vi "Main.vi"() -> ()   [LabVIEW 2018]
uses:
  cluster_enum.ctl
  Notifier_control.ctl
  <vilib>/DAQmx/configure/timing.llb/DAQmx Timing (Sample Clock).vi
  <resource>/objmgr/daqmx.rc
panel:
  in  "C Module":T1=enum."Strain Card 1 Tared"
  in  "Stop 4":bool caption="Stop"
  in  "Card 2 Samples Per Loop":i32=100 caption="Numeric"
  in  "Tab Control":enum32{"Telemetry", "DAQ Settings"}(tab)
  in  "Save":bool
  in  "Test Name":string caption="String"
  out "Accel Card Rate":dbl caption="Numeric"
  in  "Card 2 Sample Rate Setpoint":dbl=100.0 caption="Numeric"
  in  "Card 1 Rate Setpoint":dbl=1000.0 caption="Numeric"
  out "Strain Card 1 Rate":dbl caption="Numeric"
  in  "Card 1 Samples Per Loop":i32=100 caption="Numeric"
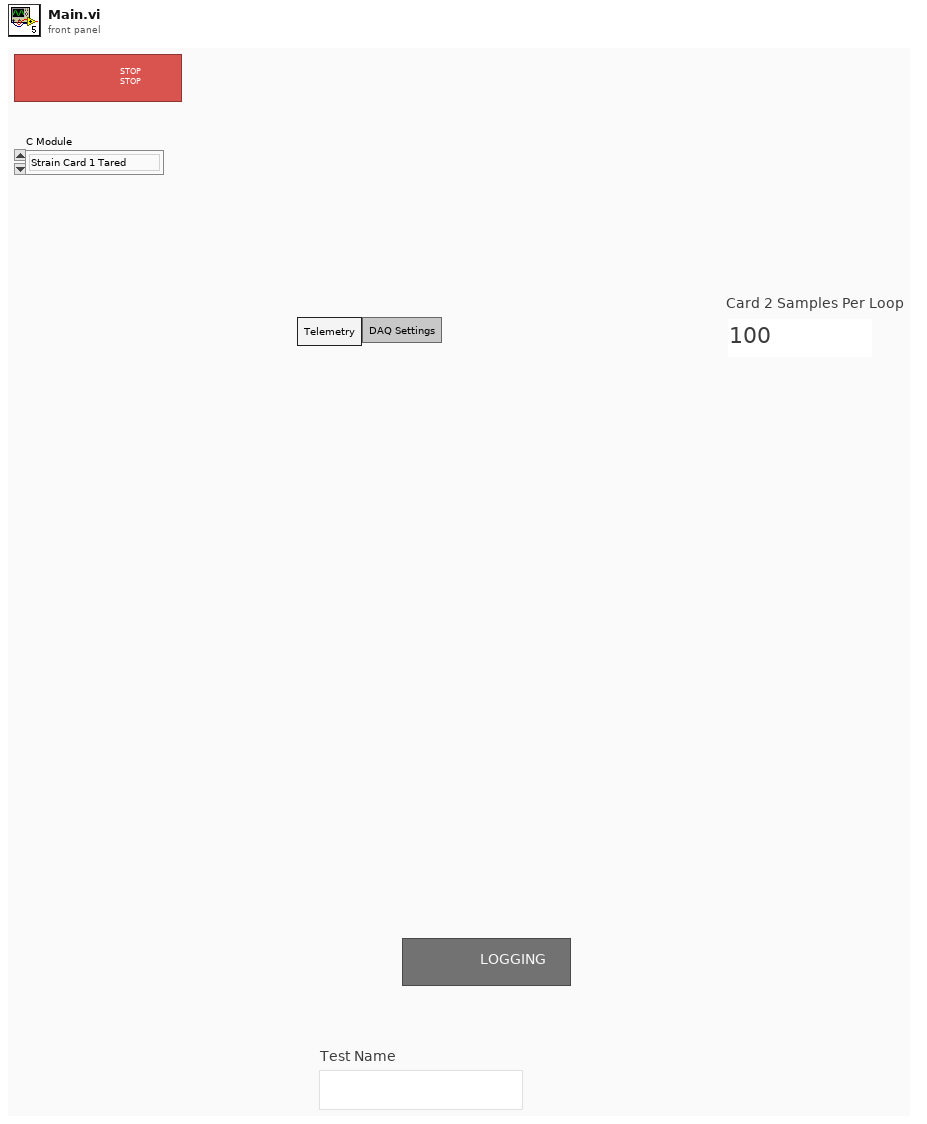
[diagram p1: front panel]
types:
  T1 = typedef "cluster_enum.ctl" = enum16{"Strain Card 2", "Strain Card 2 Tared", "Strain Card 1 Tared", "Strain Card 1", "Accel Card 1", "Accel Card 1 Tared", ""}
  T2 = typedef "Notifier_control.ctl" = enum16{"Quit", "Run", "Save"}
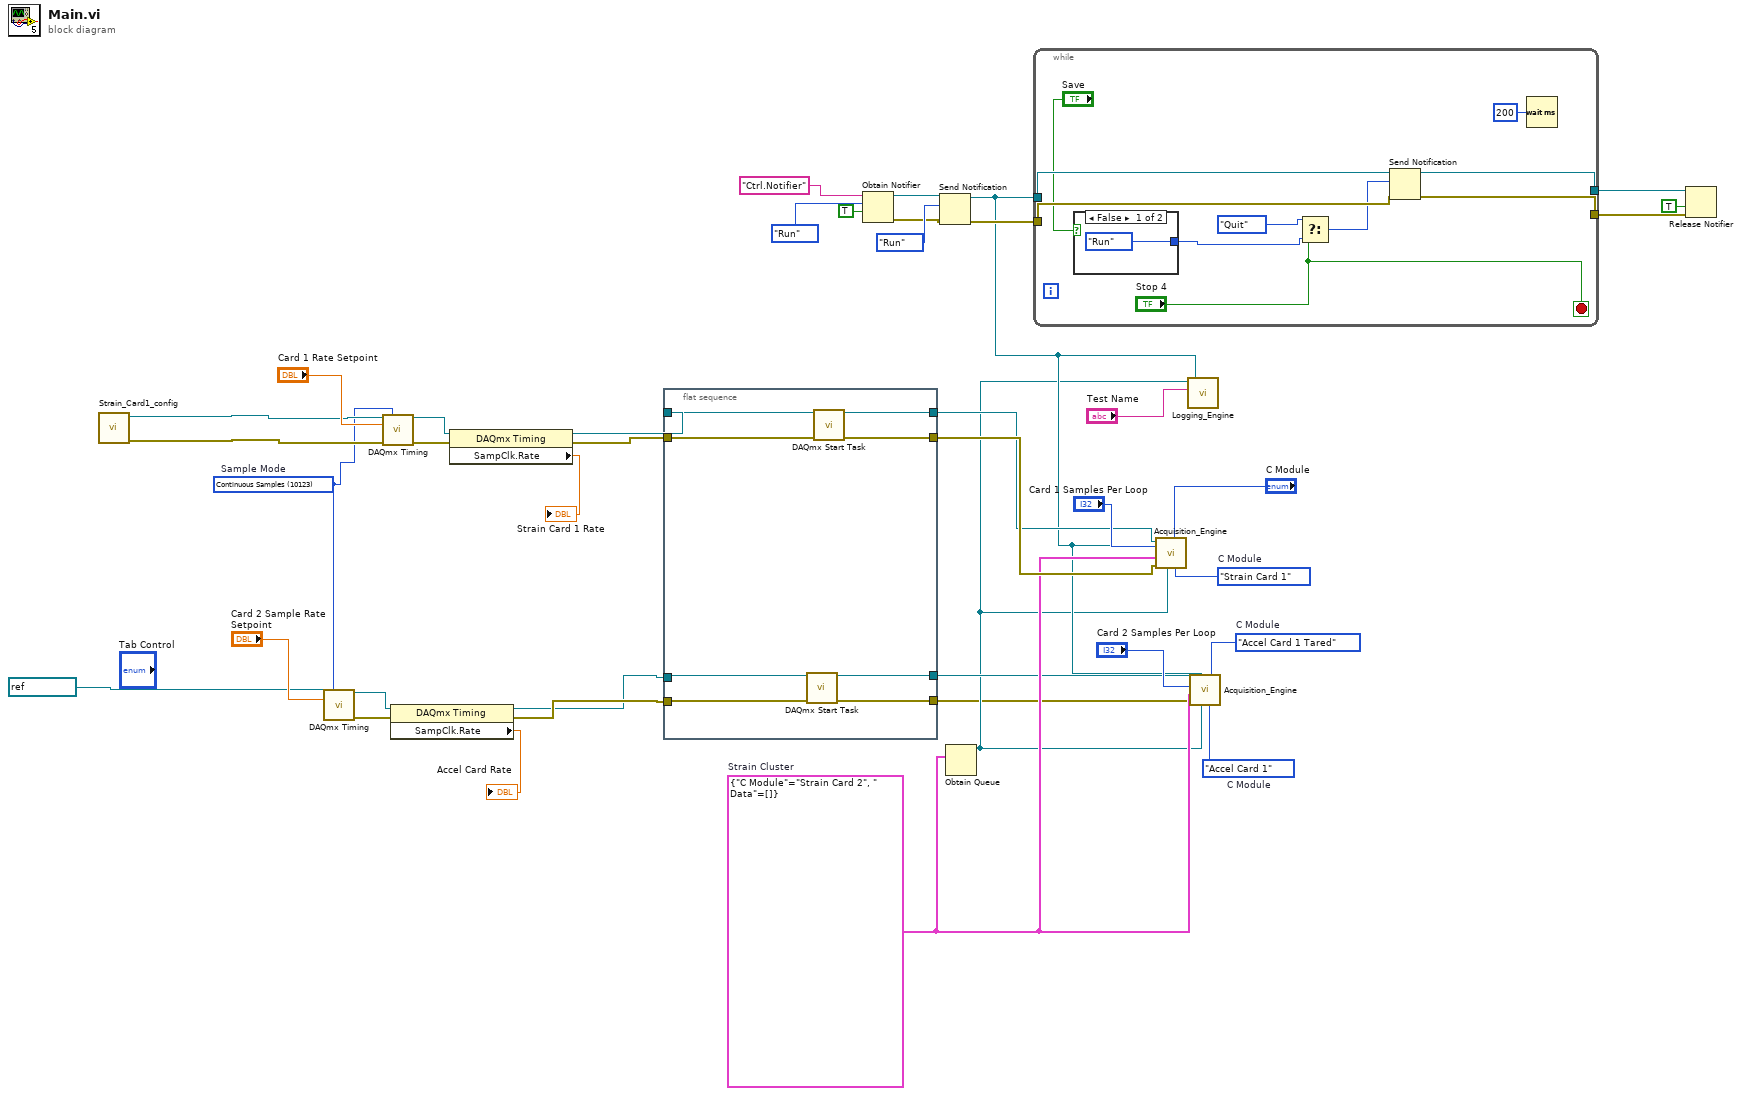
[diagram p0: block diagram]
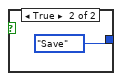
[diagram p2: hidden frame]
diagram:
  w2 = cluster_enum."Strain Card 1"  # C Module
  w3 = cluster_enum."Accel Card 1 Tared"  # C Module
  w4 = cluster_enum."Accel Card 1"  # C Module
  w10 = cluster{"C Module":T1, " Data":waveform(dbl)[]} {"C Module"=enum."Strain Card 2", " Data"=[]}  # Strain Cluster
  w26 = 10123 items=["Finite Samples"=10178, "Continuous Samples"=10123, "Hardware Timed Single Point"=12522]  # Sample Mode
  n1 = call "Strain_Card1_config.vi"() -> ("error out"=w33:errorcluster, "task out"=w34:refnum<k21>)  [unwired: 10 in]
  n2 = call-poly <vilib>:"DAQmx Timing.vi"("task/channels in"=refnum<k21> "Voltage", "sample mode"=w26, "rate"="Card 2 Sample Rate Setpoint") -> ("task out"=w32:refnum<k21>, "error out"=w31:errorcluster)  [unwired: 11 in]
  n3 = call-poly <vilib>:"DAQmx Timing.vi"("task/channels in"=w34, "sample mode"=w26, "rate"="Card 1 Rate Setpoint", "error in"=w33) -> ("task out"=w40:refnum<k21>, "error out"=w39:errorcluster)  [unwired: 10 in]
  n4 = property class="DAQmx Timing"(reference=w32, error in=w31) -> (reference out=w27:refnum<k21>, error out=w28:errorcluster, "SampClk.Rate"=→"Accel Card Rate":dbl)
  n5 = property class="DAQmx Timing"(reference=w40, error in=w39) -> (reference out=w38:refnum<k21>, error out=w37:errorcluster, "SampClk.Rate"=→"Strain Card 1 Rate":dbl)
  n6 = flat-sequence {
    tunnel: [w48] -> w22
    tunnel: w38 -> [w47]
    tunnel: w37 -> [w46]
    tunnel: [w45] -> w24
    tunnel: w28 -> [w44]
    tunnel: w27 -> [w43]
    tunnel: [w42] -> w8
    tunnel: [w41] -> w5
    frame #0 {
      n7 = call <vilib>:"DAQmx Start Task.vi"("task/channels in"=w43, "error in"=w44) -> ("task out"=w42:refnum<k21>, "error out"=w41:errorcluster)  [unwired: 12 in]
      n8 = call <vilib>:"DAQmx Start Task.vi"("task/channels in"=w47, "error in"=w46) -> ("task out"=w48:refnum<k21>, "error out"=w45:errorcluster)  [unwired: 12 in]
    }
  }
  n9 = Obtain Notifier(name (unnamed)="Ctrl.Notifier", notification data type=Notifier_control."Run", create if not found? (T)=TRUE) -> (notifier out=w17:refnum<notifier>, error out=w14:errorcluster)  [unwired: 1 in, 1 out]
  n10 = Send Notification(notification=Notifier_control."Run", notifier=w17, error in (no error)=w14) -> (notifier out=w7:refnum<notifier>, error out=w15:errorcluster)
  n11 = Obtain Queue(element data type=w10) -> (queue out=w6:refnum<queue>)  [unwired: 4 in, 2 out]
  n12 = while {
    tunnel: w7 -> [w53]
    tunnel: w15 -> [w52]
    tunnel: [w57] -> w13
    tunnel: [w56] -> w12
    stop <- "Stop 4" stop-if-true
    n13 = case shown="False" "Save" {
      tunnel: [Notifier_control."Run" Notifier_control."Save"] -> w49
      frame False {
      }
      frame True {
      }
    }
    n14 = Select(t=Notifier_control."Quit", s="Stop 4", f=w49) -> (s? t:f=w51:T2)
    n15 = Send Notification(notification=w51, notifier=w53, error in (no error)=w52) -> (notifier out=w57:refnum<notifier>, error out=w56:errorcluster)
    n16 = Wait (ms)(milliseconds to wait=u32 200) -> ()  [unwired: 1 out]
  }
  n17 = call "Acquisition_Engine.vi"("Input"=w2, "Tared Input"="C Module", "queue in"=w6, "notifier out"=w7, "DAQmx Error"=w24, "Card Cluster"=w10, "Card Samples Per Loop"="Card 1 Samples Per Loop", "task out"=w22) -> ()  [unwired: 4 in]
  n18 = call "Logging_Engine.vi"("queue out"=w6, "Test Name"="Test Name", "notifier out"=w7) -> ()  [unwired: 7 in]
  n19 = call "Acquisition_Engine.vi"("Input"=w4, "Tared Input"=w3, "queue in"=w6, "notifier out"=w7, "DAQmx Error"=w5, "Card Cluster"=w10, "Card Samples Per Loop"="Card 2 Samples Per Loop", "task out"=w8) -> ()  [unwired: 4 in]
  n20 = Release Notifier(notifier=w13, force destroy? (F)=TRUE, error in (no error)=w12) -> ()  [unwired: 3 out]
